vi "GetR.vi"(8 "error in (no error)":errorcluster, 11 "ColorRGB in":refnum<class "ColorRGB.lvclass">) -> (0 "error out":errorcluster, 2 "R":u8, 3 "ColorRGB out":refnum<class "ColorRGB.lvclass">)   [LabVIEW 2021, in "Picture2D.lvlib" / "ColorRGB.lvclass"]
uses:
  ColorRGB.lvclass
  ColorRGB.lvclass/ColorRGB.ctl
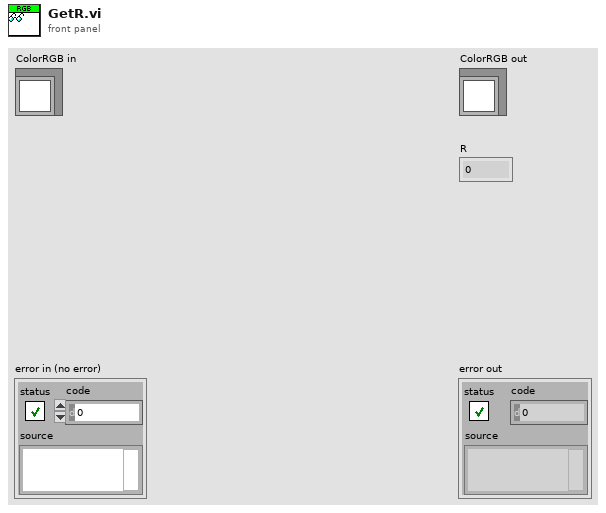
[diagram p1: front panel]
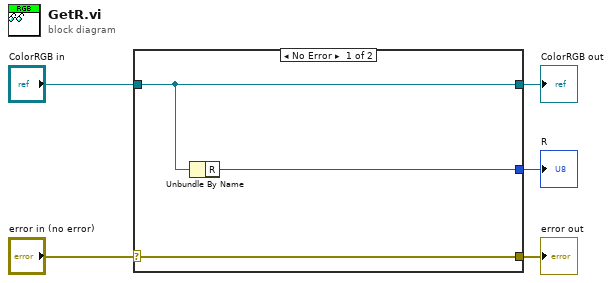
[diagram p0: block diagram]
diagram:
  n1 = case shown="No Error" "error in (no error)" {
    selector: "error in (no error)" -> [w8 w9]
    tunnel: [w8 w9] -> w4
    tunnel: [w7 w10] -> w2
    tunnel: "ColorRGB in" -> [w7 w10]
    tunnel: [w6 _] -> w1
    frame No Error {
      n2 = Unbundle By Name(w7) -> ("R"=w6:u8)
    }
    frame Error {
    }
  }
  "error out" <- w4
  "ColorRGB out" <- w2
  "R" <- w1
